vi "Enable square wave.vi"(8 "Error In":errorcluster, 10 "Enable wave":bool, 11 "Arduino port in":refnum<visa-resource-name>) -> (0 "Error Out":errorcluster, 3 "Arduino port out":refnum<visa-resource-name>)   [LabVIEW 2016]
uses:
  Typedef/AD5535 - Command.ctl
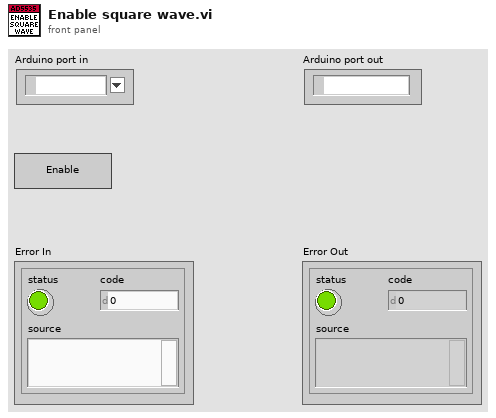
[diagram p1: front panel]
types:
  T1 = typedef "AD5535 - Command.ctl" = enum16{"None", "Start", "Stop", "Load Array", "Update channel", "Update frequency", "Prova"}
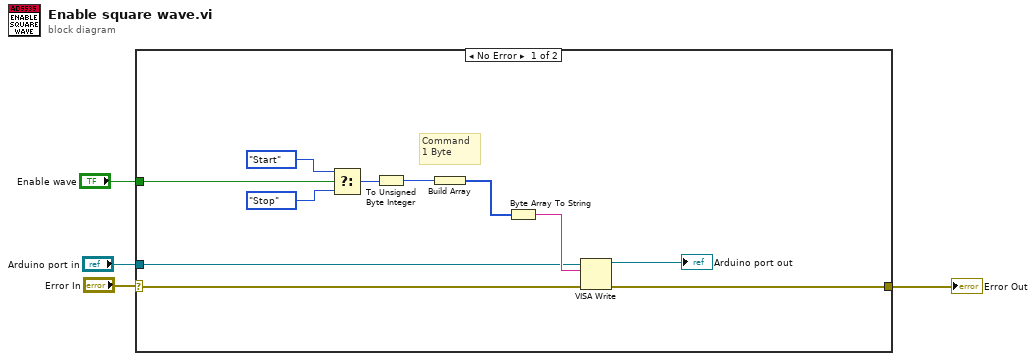
[diagram p0: block diagram]
diagram:
  n1 = case shown="No Error" "Error In" {
    selector: "Error In" -> [w15 w16]
    tunnel: [w14 w16] -> w2
    tunnel: "Arduino port in" -> [w12 _]
    tunnel: "Enable wave" -> [w8 _]
    frame No Error {
      # "Command\n1 Byte"
      n2 = Select(t=AD5535_-_Command."Start" ("AD5535 - Command"), s=w8, f=AD5535_-_Command."Stop" ("AD5535 - Command")) -> (s? t:f=w5:T1)
      n3 = To Unsigned Byte Integer(number=w5) -> (unsigned 8bit integer=w11:u8)
      n4 = Build Array(w11) -> (w10:u8[])
      n5 = Byte Array To String(unsigned byte array=w10) -> (string=w13:string)
      n6 = VISA Write(VISA resource name=w12, write buffer=w13, error in (no error)=w15) -> (VISA resource name out=→"Arduino port out":refnum<visa-resource-name>, error out=w14:errorcluster)  [unwired: 1 out]
    }
    frame Error {
    }
  }
  "Error Out" <- w2
